vi "START3FLOWRATEGOOD.vi"() -> ()   [LabVIEW 2024]
uses:
  <vilib>/Utility/file.llb/Read Delimited Spreadsheet (DBL).vi
panel:
  out "LVAD Speed Waveform":dbl[](graph)
  out "Flow Rate Waveform":dbl[](graph)
  in  "stop":bool
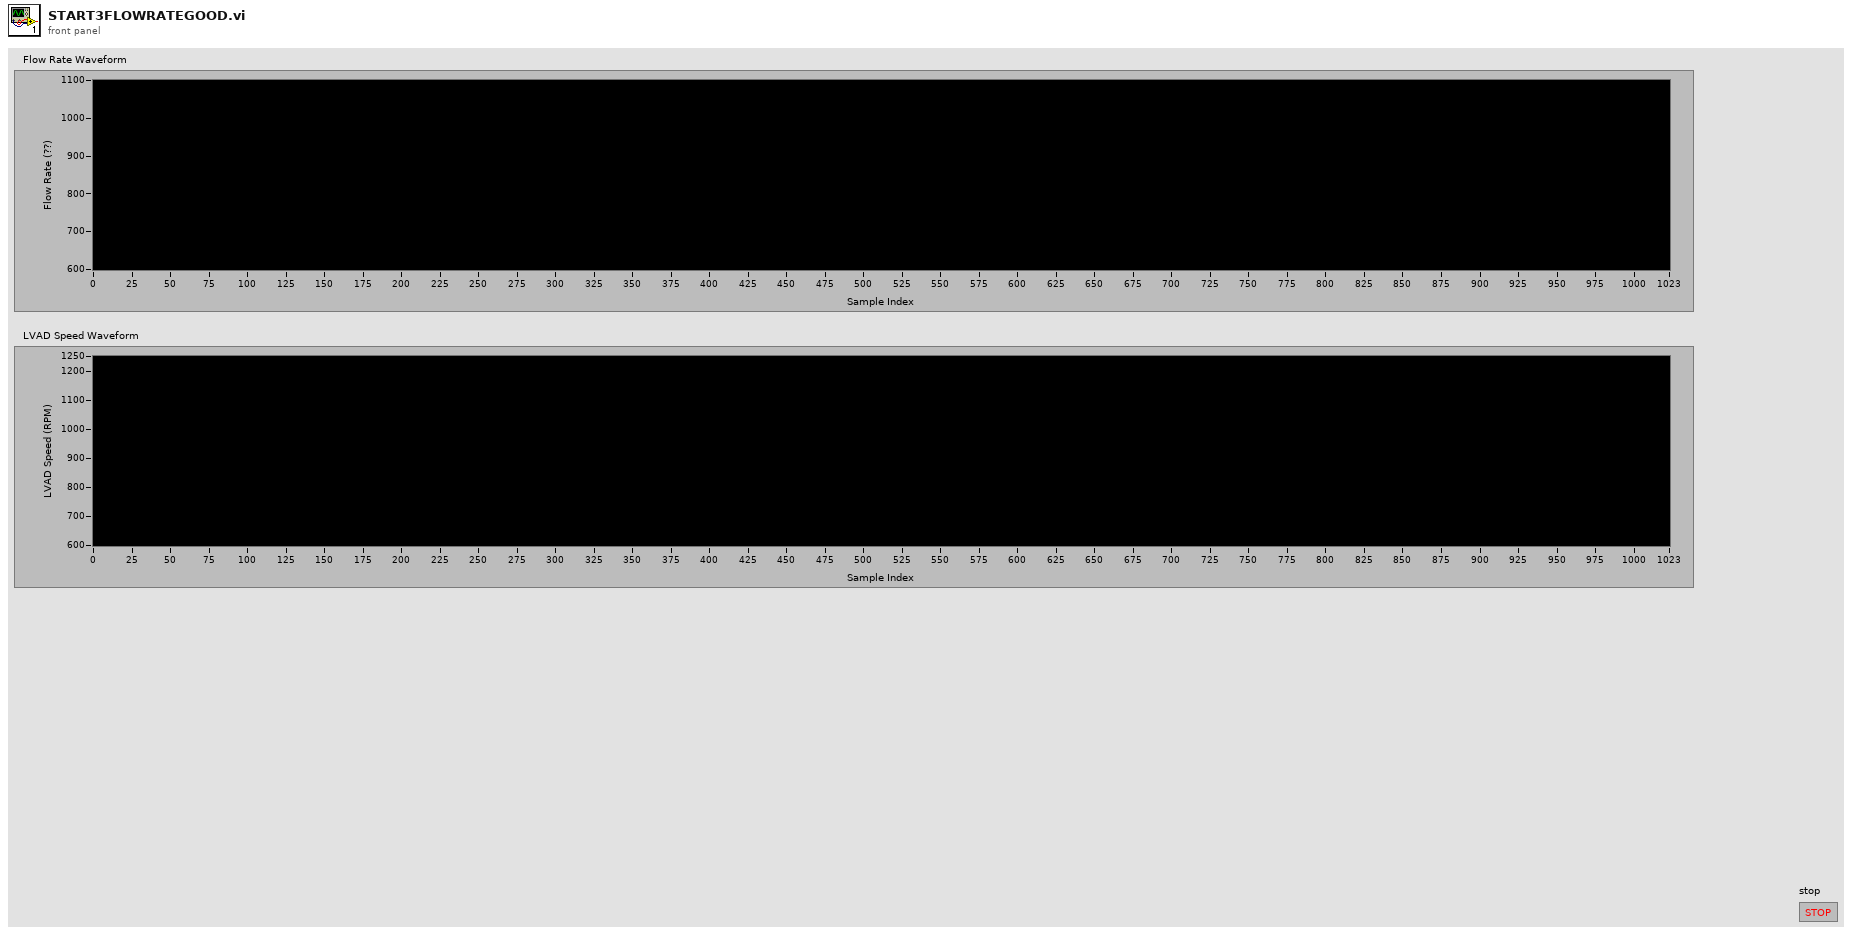
[diagram p1: front panel]
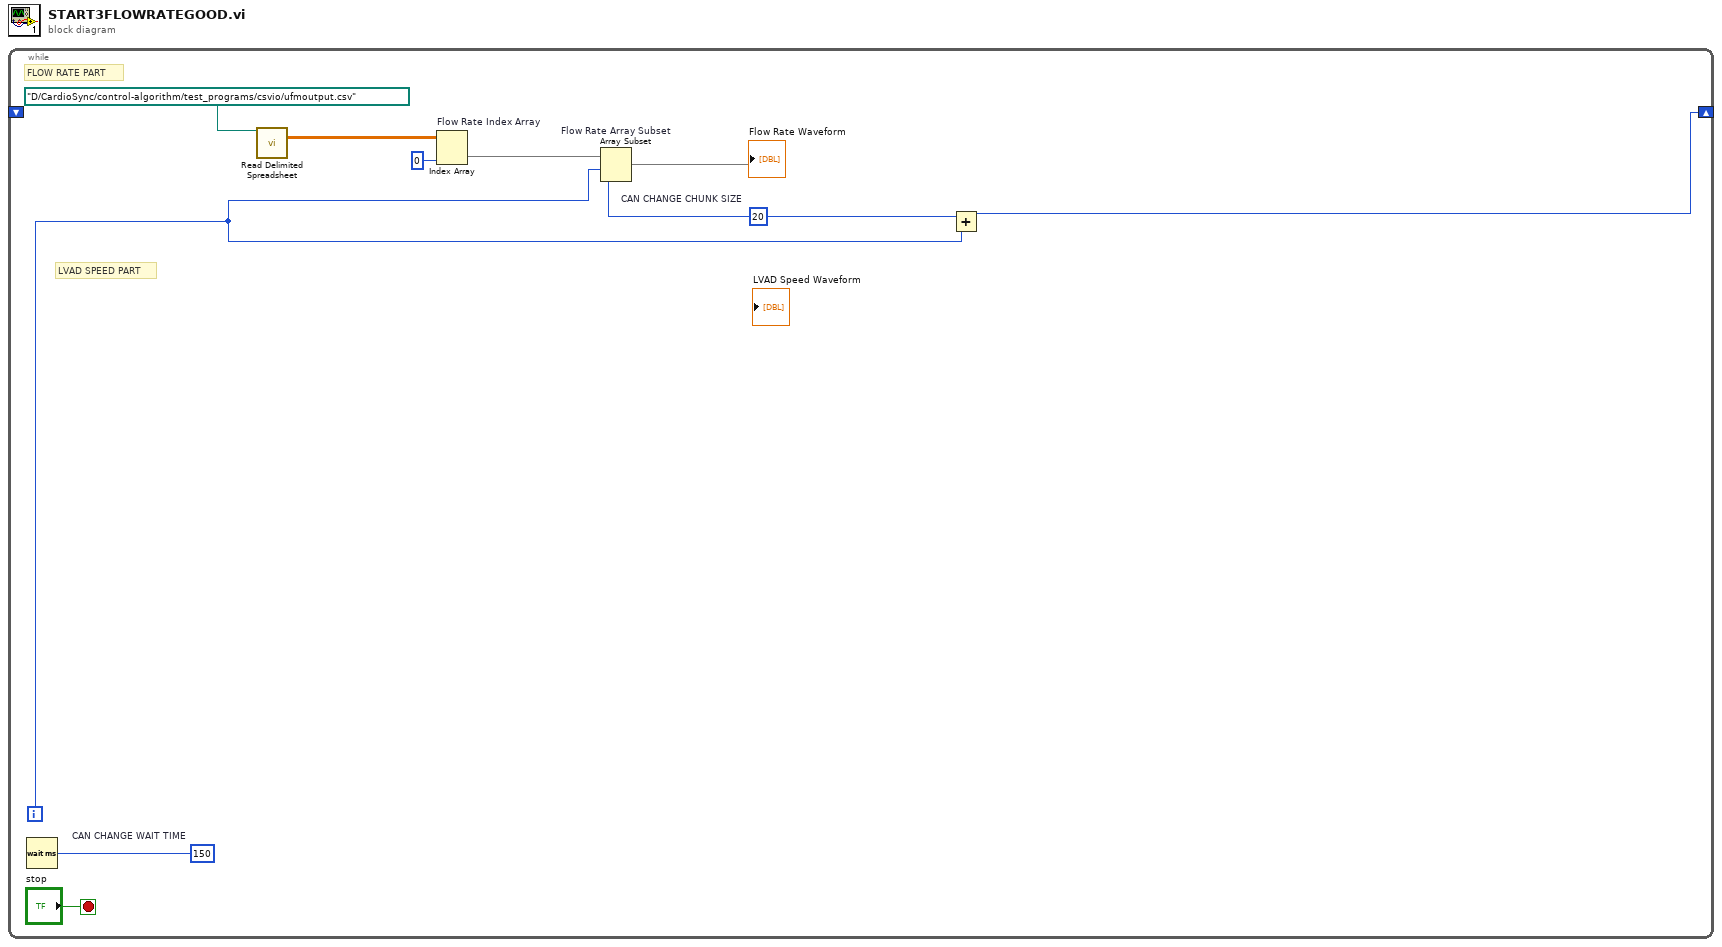
[diagram p0: block diagram]
diagram:
  n1 = while {
    shift-right: [w5] -> _
    shift-left: _ -> [_]
    i -> [w2]
    stop <- "stop" stop-if-true
    w6 = u32 150  # CAN CHANGE WAIT TIME
    w3 = 20  # CAN CHANGE CHUNK SIZE
    # "LVAD SPEED PART"
    # "FLOW RATE PART"
    n2 = Wait (ms)(milliseconds to wait=w6) -> ()  [unwired: 1 out]
    n3 = call-poly <vilib>:"Read Delimited Spreadsheet.vi"("file path (dialog if empty)"=path "D:/CardioSync/control-algorithm/test_programs/csvio/ufmoutput.csv") -> ("all rows"=w8:dbl[][])  [unwired: 9 in, 5 out]
    n4 = Index Array "Flow Rate Index Array"(array=w8, index (col)=0 ("disabled index (col)")) -> (element=w7:dbl[])  [unwired: 1 in]
    n5 = Array Subset "Flow Rate Array Subset"(array=w7, index=w2, length=w3) -> (→"Flow Rate Waveform":dbl[])
    n6 = Add(x=w3, y=w2) -> (x+y=w5:i32)
  }
